vi "red.vi"(0 "Image In":T2, 1 "Red BCG Values (Brightness 1)":T1={"Brightness"=255.0, "Contrast"=89.0, "Gamma"=0.14468643}, 2 "Green BCG Values (Brightness 1)":T1={"Brightness"=255.0, "Contrast"=78.23404, "Gamma"=10.0}, 3 "Blue BCG Values (Brightness 1)":T1={"Brightness"=255.0, "Contrast"=78.23404, "Gamma"=10.0}, 7 "error in":errorcluster) -> (20 "Image Out":T2, 27 "error out":errorcluster)   [LabVIEW 2020]
uses:
  <vilib>/vision/Image Controls.llb/IMAQ Image.ctl
  <vilib>/vision/NI_Vision_Development_Module.lvlib
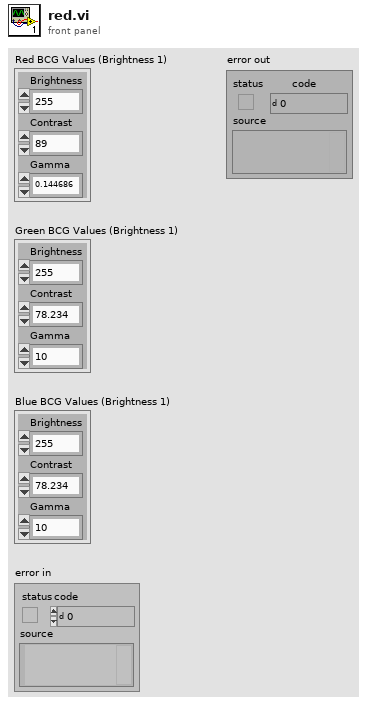
[diagram p1: front panel]
types:
  T1 = cluster{"Brightness":sgl, "Contrast":sgl, "Gamma":sgl}
  T2 = typedef "IMAQ Image.ctl" = refnum<image>
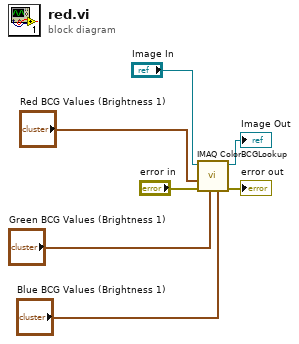
[diagram p0: block diagram]
diagram:
  n1 = call "IMAQ ColorBCGLookup"("Blue BCG Values"="Blue BCG Values (Brightness 1)", "Green BCG Values"="Green BCG Values (Brightness 1)", "error in (no error)"="error in", "Red BCG Values"="Red BCG Values (Brightness 1)", "Image Src"="Image In") -> ("error out"=→"error out":errorcluster, "Image Dst Out"=→"Image Out":T2)  [unwired: 2 in, 3 out]
